vi "SftpCreateDirectory.vi"(0 "error in":errorcluster, 7 "Robot Path":string, 11 "Sftp":refnum<k24>) -> (4 "error out":errorcluster)   [LabVIEW 2022 SP3, in "UnderAutomation.UniversalRobots.lvlib"]
uses:
  UnderAutomation.UniversalRobots.lvlib
  C:/Users/fg/Documents/UniversalRobots.vi/LabVIEW_2024/UnderAutomation.UniversalRobots/lib/UnderAutomation.UniversalRobots.dll
  LabVIEW_2024/UnderAutomation.UniversalRobots/lib/UnderAutomation.UniversalRobots.dll
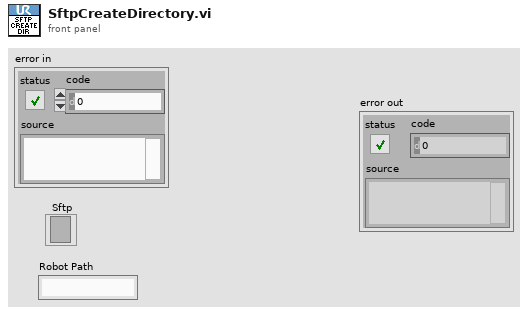
[diagram p1: front panel]
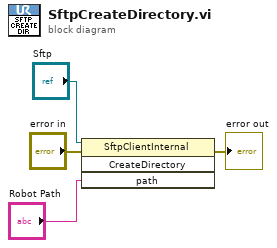
[diagram p0: block diagram]
diagram:
  n1 = invoke class="SftpClientInternal" method="CreateDirectory"(reference="Sftp", error in="error in", "path"="Robot Path") -> (error out=→"error out":errorcluster)  [unwired: 1 in, 3 out]
